vi "Do.vi"(8 "error in (no error)":errorcluster, 10 "Actor in":refnum<class "Actor.lvclass">, 11 "Conceret Test Node Map Msg":refnum<class "Conceret Results Msg.lvclass">) -> (0 "error out":errorcluster, 2 "Actor out":refnum<class "Actor.lvclass">)   [LabVIEW 2013, in "Hot And Cold Source Unit View.lvlib" / "Conceret Results Msg.lvclass"]
doc: "(<B>Filename</B>: Actor Framework.lvlib:Message.lvclass:Do.vi)\n\nDefines what a message does when it is received by an actor. Generally, a message instructs an actor to invoke one of its methods.\n\nBy default, this method does nothing. A child class must override it to define behavior. Create a child class by using the Actor Framework Message Maker dialog box."
uses:
  Conceret Results Msg.lvclass
  <vilib>/ActorFramework/Actor/Actor.lvclass
  Views/Hot And Cold Source Unit View/Hot And Cold Source Unit View.lvclass
  Abstract Results Msg/Abstract Results Msg.lvclass
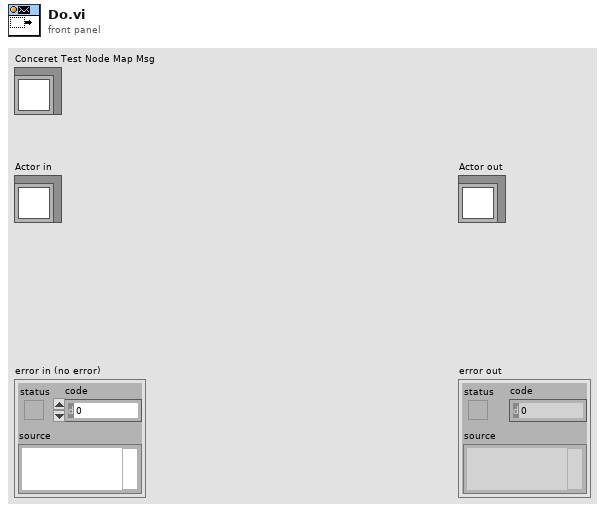
[diagram p1: front panel]
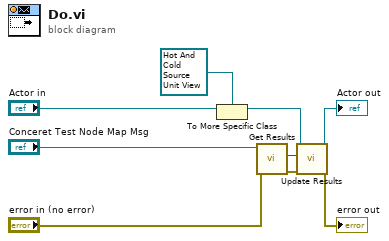
[diagram p0: block diagram]
diagram:
  n1 = To More Specific Class(target class=refnum<class "Hot And Cold Source Unit View.lvclass"> refnum ("Hot And Cold Source Unit View.lvlib:Hot And Cold Source Unit View.lvclass"), reference="Actor in") -> (specific class reference=w8:refnum<class "Hot And Cold Source Unit View.lvclass">)  [unwired: 1 in, 1 out]
  n2 = call "Get Results.vi"("error in (no error)"="error in (no error)", "Abstract Results Msg in"="Conceret Test Node Map Msg") -> ("error out"=w7:errorcluster, "Results"=w6:variant)  [unwired: 7 in, 1 out]
  n3 = call "Update Results.vi"("error in (no error)"=w7, "Results"=w6, "Hot And Cold Source Unit View in"=w8) -> ("error out"=→"error out":errorcluster, "Hot And Cold Source Unit View out"=→"Actor out":refnum<class "Hot And Cold Source Unit View.lvclass">)  [unwired: 7 in]
